vi "Draw XY Projection Read.vi"(4 "error in (no error)":errorcluster, 6 "Container State":T3, 7 "Display State In":T1) -> (0 "error out":errorcluster, 2 "Value":bool, 3 "Display State Out":T1)   [LabVIEW 2020, in "3D Comet.xctl"]
uses:
  <vilib>/Math Plots/3D Math Plots/3D Comet/3D Comet XCtrl/3D Comet.xctl
  <vilib>/_xctls/Container State.ctl
  <vilib>/Math Plots/3D Math Plots/3D Comet/3D Comet XCtrl/State.ctl
  <vilib>/Math Plots/3D Math Plots/3D Comet/3D Comet/3D Comet.lvclass
  e:/builds/penguin/labview/branches/2020/dev/dist/vi.lib/Math Plots/3D Math Plots/3D Plot/3D Plot/3D Plot.lvclass
  <vilib>/Math Plots/3D Math Plots/3D Plot/Action String/3DMathPlot Ctrl Act Queue.ctl
  <vilib>/Math Plots/3D Math Plots/3D Plot/Action String/3DMathPlot Ctrl Act Cluster.ctl
  <vilib>/Math Plots/3D Math Plots/3D Plot/Action String/3DMathPlot State Class.ctl
  <vilib>/Math Plots/3D Math Plots/3D Plot/3D Plot/3D Plot.lvclass
  <vilib>/_xctls/XControlSupport.lvlib
panel:
  # "Replace the Value Indicator below with an Indicator of desired type.\nDo not remove this Indicator or the others from the connector pane. \nDo not change the connector pane pattern.\nThe Value Indicator should always be the second terminal from top on the output side in the connector pane."
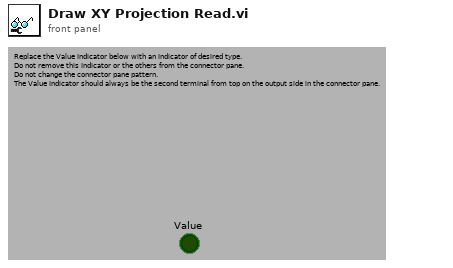
[diagram p1: front panel]
types:
  T1 = typedef "3D Comet.xctl/State.ctl" = cluster{"3D Comet.lvclass":refnum<class "3D Comet.lvclass">, "Control Ref Queue":T2, "Main Frame Color":u32, "Ramp Palette Color":u32, "Projection Palette Color":u32}
  T2 = typedef "3DMathPlot Ctrl Act Queue.ctl" = refnum<queue>
  T3 = typedef "XControlSupport.lvlib/Container State.ctl" = cluster{"Indicator?":bool, "Run Mode?":bool, " Refnum":refnum<vi>}
  T4 = typedef "3D Comet.lvclass/3D Comet Property Array.ctl" = T5[]
  T5 = typedef "3D Comet.lvclass/3D Comet Property.ctl" = cluster{"General Property":cluster{"Plot Name":string, "Coordinate System":enum16{"Cartesian", "Cylindrical", "Spherical"}, "Opacity":sgl}, "Projection Property":cluster{"Draw XY":bool, "Draw YZ":bool, "Draw XZ":bool}, "Plot Property":cluster{"Sprite Type":T6, "Point Size":sgl, "Point Color":u32, "Line Style":T7, "Line Width":sgl, "Line Color":u32, "Antialiasing":bool}, "Comet Property":cluster{"Body length":sgl}}
  T6 = typedef "3D Plot.lvclass/Sprite Type.ctl" = enum16{"None", "Empty Square", "Solid Square", "Empty Diamond", "Solid Diamond", "Empty Circle", "Solid Circle", "Asterisk", "Bold X", "Wireframe Sphere", "Solid Sphere", "Wireframe Cube", "Solid Cube"}
  T7 = typedef "3D Plot.lvclass/Line Type.ctl" = enum16{"None", "Solid", "Dash", "Dot", "Dash Dot"}
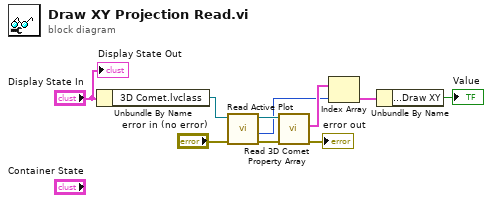
[diagram p0: block diagram]
diagram:
  n1 = Unbundle By Name("Display State In") -> ("3D Comet.lvclass"=w9:refnum<class "3D Comet.lvclass">)
  n2 = call <vilib>:"Read Active Plot.vi"("error in (no error)"="error in (no error)", "3D Plot.lvclass in"=w9) -> ("error out"=w6:errorcluster, "Active Plot"=w5:i32, "3D Plot.lvclass out"=w8:refnum<class "3D Comet.lvclass">)  [unwired: 7 out]
  n3 = call <vilib>:"Read 3D Comet Property Array.vi"("error in (no error)"=w6, "3D Comet.lvclass in"=w8) -> ("error out"=→"error out":errorcluster, "3D Comet Property Array"=w7:T4)  [unwired: 8 out]
  n4 = Index Array(array=w7, index=w5) -> (element=w10:T5)
  n5 = Unbundle By Name(w10) -> ("Projection Property.Draw XY"=→"Value":bool)
  "Display State Out" <- "Display State In"
